vi "read_MonitorGain.vi"() -> ()   [LabVIEW 2014]
uses:
  aardvark.dll
panel:
  out "Gain":dbl
  in  "Address (0x50)":u16=80 max=1023 format="%.0x"
  in  "Num Bytes to Fetch (64)":u8=64 min=1
  in  "Aardvark Handle":i32 min=0
  in  "error in (no error)":errorcluster
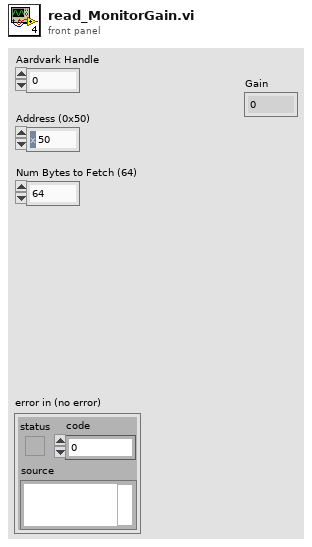
[diagram p1: front panel]
types:
  T1 = cluster{"unsigned byte array[0]":u8, "unsigned byte array[1]":u8, "unsigned byte array[2]":u8, "unsigned byte array[3]":u8, "unsigned byte array[4]":u8, "unsigned byte array[5]":u8, "unsigned byte array[6]":u8, "unsigned byte array[7]":u8, "unsigned byte array[8]":u8}
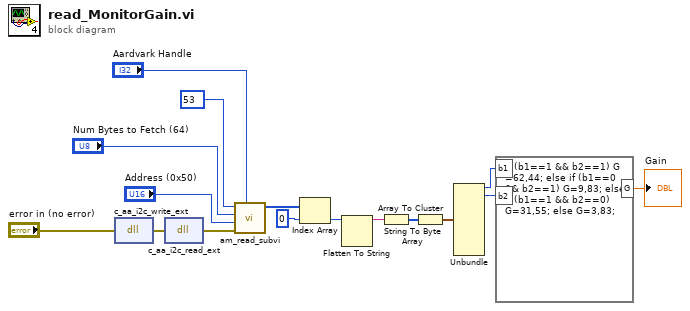
[diagram p0: block diagram]
diagram:
  n1 = dll-call lib="C:/Users/p282652/Documents/LabVIEW Data/Demonstrator/labviewFunctions_AM/aardvark.dll" fn="c_aa_i2c_write_ext"(error in="error in (no error)") -> (error out=w7:errorcluster)  [unwired: 3 in, 1 out]
  n2 = dll-call lib="C:/Users/p282652/Documents/LabVIEW Data/Demonstrator/labviewFunctions_AM/aardvark.dll" fn="c_aa_i2c_read_ext"(error in=w7) -> (error out=w6:errorcluster)  [unwired: 3 in, 1 out]
  n3 = call "am_read_subvi.vi"("Aardvark Handle in"="Aardvark Handle", "error in (no error)"=w6, "Address (0x50) in"="Address (0x50)", "Num Bytes to Fetch (64)"="Num Bytes to Fetch (64)", "Memory ADD"=u16 53) -> ("Array"=w1:u8[])  [unwired: 5 in, 1 out]
  n4 = Index Array(array=w1, index=0) -> (element=w12:u8)
  n5 = Flatten To String(anything=w12) -> (data string=w15:string)  [unwired: 3 in, 2 out]
  n6 = String To Byte Array(string=w15) -> (unsigned byte array=w14:u8[])
  n7 = Array To Cluster(array=w14) -> (cluster=w13:T1)
  n8 = Unbundle(w13) -> ("unsigned byte array[0]"=w11:u8, "unsigned byte array[1]"=w10:u8)  [unwired: 7 out]
  n9 = formula code="if (b1==1 && b2==1) G =62,44; else if (b1==0 && b2==1) G=9,83; else if (b1==1 && b2==0) G=31,55; else G=3,83;"("b1"=w11, "b2"=w10) -> ("G"=→"Gain":dbl)
